vi "think.vi"(0 "X":i8, 1 "Y":i8, 2 "Sensor Array":i8[][](array[numeric]), 3 "Sense Heading":i8, 4 "E":i8) -> (5 "V Heading":i8)   [LabVIEW 2012]
doc: "Chooses a direction of travel based on the direction to the highest-valued block in the world at a given moment. These values are assigned based on known food locations, potential food locations, and proximity to the current robot location."
panel:
  out "Tan":dbl
  out "Expected Value":dbl[][](array[numeric])
  out "Robot Memory":i8[][](array[numeric])
  # "World Key\n-1 = not visited\n0 = no food\n[1...] = food"
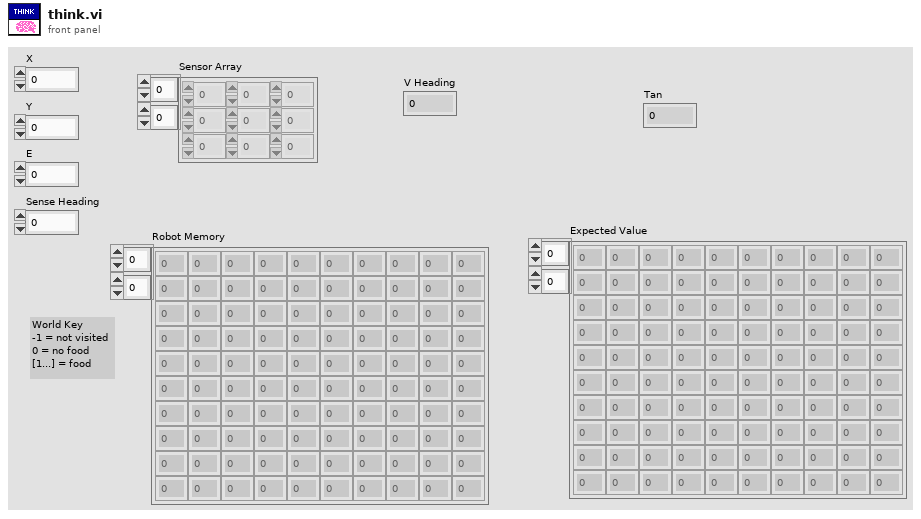
[diagram p1: front panel]
types:
  T1 = cluster{"[0]":i32, "[1]":i32, "[2]":i32, "[3]":i32, "[4]":i32, "[5]":i32, "[6]":i32, "[7]":i32, "[8]":i32}
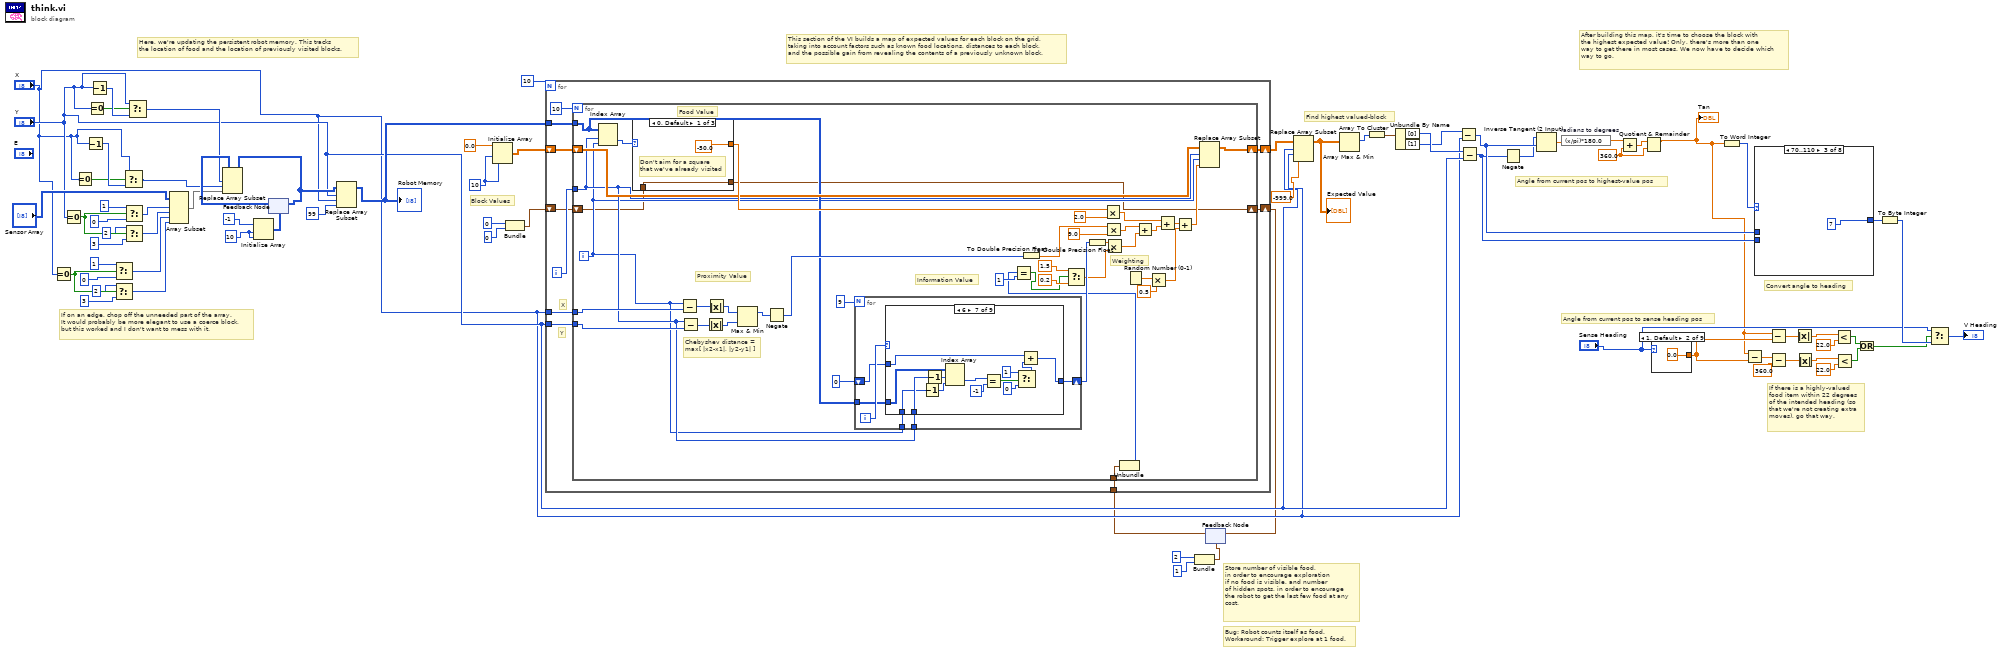
[diagram p0: block diagram]
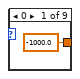
[diagram p2: hidden frame]
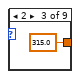
[diagram p3: hidden frame]
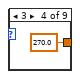
[diagram p4: hidden frame]
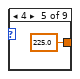
[diagram p5: hidden frame]
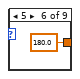
[diagram p6: hidden frame]
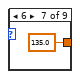
[diagram p7: hidden frame]
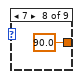
[diagram p8: hidden frame]
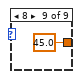
[diagram p9: hidden frame]
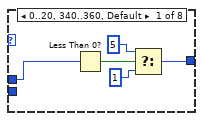
[diagram p10: hidden frame]
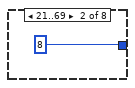
[diagram p11: hidden frame]
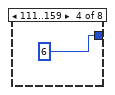
[diagram p12: hidden frame]
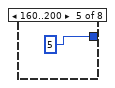
[diagram p13: hidden frame]
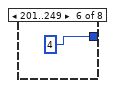
[diagram p14: hidden frame]
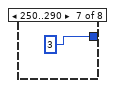
[diagram p15: hidden frame]
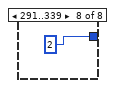
[diagram p16: hidden frame]
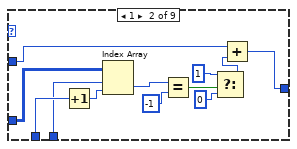
[diagram p18: hidden frame]
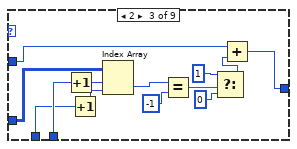
[diagram p19: hidden frame]
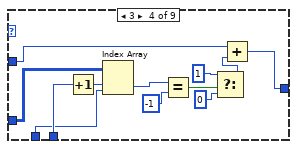
[diagram p20: hidden frame]
diagram:
  w31 = 360.0
  w44 = 10
  w74 = 10
  # "If there is a highly-valued\nfood item within 22 degrees\nof the intended heading (so\nthat we're not creating extra\nmoves), go that way."
  # "Angle from current pos to sense heading pos"
  # "Angle from current pos to highest-value pos"
  # "Convert angle to heading"
  # "Bug: Robot counts itself as food.\nWorkaround: Trigger explore at 1 food."
  # "Store number of visible food,\nin order to encourage exploration\nif no food is visible, and number\nof hidden spots, in order to encourage\nthe robot to get the last few food at any\ncost."
  # "Find highest valued-block"
  # "Here, we're updating the persistent robot memory. This tracks\nthe location of food and the location of previously visited blocks."
  # "After building this map, it's time to choose the block with\nthe highest expected value! Only, there's more than one\nway to get there in most cases. We now have to decide which\nway to go."
  # "This section of the VI builds a map of expected values for each block on the grid, \ntaking into account factors such as known food locations, distances to each block,\nand the possible gain from revealing the contents of a previously unknown block."
  # "Block Values"
  # "If on an edge, chop off the unneeded part of the array.\nIt would probably be more elegant to use a coerce block,\nbut this worked and I don't want to mess with it."
  n1 = Equal To 0?(x="X") -> (x = 0?=w69:bool)
  n2 = Equal To 0?(x="Y") -> (x = 0?=w62:bool)
  n3 = Equal To 0?(x="X") -> (x = 0?=w52:bool)
  n4 = Decrement(x="X") -> (x-1=w53:i8)
  n5 = Equal To 0?(x="Y") -> (x = 0?=w51:bool)
  n6 = Decrement(x="Y") -> (x-1=w55:i8)
  n7 = Select(t=1, s=w69, f=0) -> (s? t:f=w68:i32)
  n8 = Select(t=2, s=w69, f=3) -> (s? t:f=w67:i32)
  n9 = Select(t="X", s=w52, f=w53) -> (s? t:f=w50:i8)
  n10 = Select(t=1, s=w62, f=0) -> (s? t:f=w57:i32)
  n11 = Select(t=2, s=w62, f=3) -> (s? t:f=w56:i32)
  n12 = Select(t="Y", s=w51, f=w55) -> (s? t:f=w54:i8)
  n13 = Array Subset(array="Sensor Array", index (row)=w57, length (row)=w56, index (col)=w68, length (col)=w67) -> (w71:i8[][])
  n14 = Initialize Array(i8 -1, w74, w74) -> (w73:i8[][])
  n15 = feedback #1(w73) -> (w72:i8[][])
  n16 = Replace Array Subset(array=w72, new element=w71, index (row)=w54, index (col)=w50) -> (w49:i8[][])
  n17 = feedback-in #1(w49) -> ()
  n18 = Replace Array Subset(array=w49, new element=i8 99, index (row)="Y", index (col)="X") -> (w47:i8[][])
  "Robot Memory" <- w47
  n19 = Initialize Array(0.0, w44, w44) -> (w46:dbl[][])
  n20 = Bundle(0, 0) -> (w17:cluster{i32, i32})  [unwired: 1 in]
  n21 = Bundle(2, 1) -> (w21:cluster{i32, i32})  [unwired: 1 in]
  n22 = feedback #2(w21) -> (w24:cluster{i32, i32})
  n23 = for {
    N: 10 -> [_]
    tunnel: w47 -> [w85]
    shift-right: [w83] -> w38
    shift-left: w46 -> [w84]
    tunnel: "Y" -> [w80]
    tunnel: "X" -> [w79]
    shift-right: [w77] -> w23
    shift-left: w17 -> [w78]
    tunnel: w24 -> [w76]
    i -> [w81]
    # "Y"
    # "X"
    n24 = for {
      N: 10 -> [_]
      tunnel: w85 -> [w109]
      shift-right: [w121] -> w83
      shift-left: w84 -> [w119]
      tunnel: w81 -> [w102]
      tunnel: w80 -> [w107]
      tunnel: w79 -> [w108]
      shift-right: [w99] -> w77
      shift-left: w78 -> [w100]
      tunnel: w76 -> [w87]
      i -> [w101]
      # "Chebyshev distance =\nmax[ |x2-x1|, |y2-y1| ]"
      # "Information Value"
      # "Weighting"
      # "Proximity Value"
      # "Food Value"
      n25 = Index Array(array=w109, index (row)=w102, index (col)=w101) -> (element=w125:i8)
      n26 = case shown="0, Default" w125 {
        selector: w125 -> [_ w240 _]
        tunnel: [-50.0 w241 0.5] -> w122
        tunnel: w100 -> [w233 w238 w245]
        tunnel: [w233 w239 w246] -> w99
        frame 0, Default {
          # "Don't aim for a square\nthat we've already visited"
        }
        frame 1.. {
          n27 = Unbundle(w238) -> (w236:i32, w235:i32)
          n28 = Increment(x=w236) -> (x+1=w237:i32)
          n29 = To Double Precision Float(number=w240) -> (double precision float=w241:dbl)
          n30 = Bundle(w237, w235) -> (w239:cluster{i32, i32})  [unwired: 1 in]
        }
        frame -1 {
          n31 = Unbundle(w245) -> (w242:i32, w243:i32)
          n32 = Increment(x=w243) -> (x+1=w244:i32)
          n33 = Bundle(w242, w244) -> (w246:cluster{i32, i32})  [unwired: 1 in]
        }
      }
      n34 = Subtract(x=w101, y=w108) -> (x-y=w118:i32)
      n35 = Subtract(x=w102, y=w107) -> (x-y=w117:i32)
      n36 = Absolute Value(x=w117) -> (abs(x)=w116:i32)
      n37 = Absolute Value(x=w118) -> (abs(x)=w115:i32)
      n38 = Max & Min(x=w115, y=w116) -> (max(x,y)=w114:i32)  [unwired: 1 out]
      n39 = Negate(x=w114) -> (-x=w112:i32)
      n40 = for {
        N: 9 -> [_]
        shift-right: [w129] -> w103
        shift-left: 0 -> [w130]
        tunnel: w109 -> [w128]
        tunnel: w101 -> [w127]
        tunnel: w102 -> [w126]
        i -> [w131]
        n41 = case shown="6" w131 {
          tunnel: w130 -> [w132 w142 w155 w167 w180 w192 w205 w217 w230]
          tunnel: [w132 w141 w154 w166 w179 w191 w204 w216 w229] -> w129
          tunnel: w128 -> [_ w144 w157 w169 w182 w194 w207 w219 w232]
          tunnel: w127 -> [_ w134 w145 w158 w172 w184 w197 w208 w221]
          tunnel: w126 -> [_ w133 w146 w160 w170 w183 w198 w209 w223]
          frame 0, Default {
          }
          frame 1 {
            n42 = Increment(x=w134) -> (x+1=w135:i32)
            n43 = Index Array(array=w144, index (row)=w133, index (col)=w135) -> (element=w137:i8)
            n44 = Equal?(x=w137, y=i8 -1) -> (x = y?=w138:bool)
            n45 = Select(t=1, s=w138, f=0) -> (s? t:f=w143:i32)
            n46 = Add(x=w142, y=w143) -> (x+y=w141:i32)
          }
          frame 2 {
            n47 = Increment(x=w146) -> (x+1=w147:i32)
            n48 = Increment(x=w145) -> (x+1=w148:i32)
            n49 = Index Array(array=w157, index (row)=w147, index (col)=w148) -> (element=w150:i8)
            n50 = Equal?(x=w150, y=i8 -1) -> (x = y?=w151:bool)
            n51 = Select(t=1, s=w151, f=0) -> (s? t:f=w156:i32)
            n52 = Add(x=w155, y=w156) -> (x+y=w154:i32)
          }
          frame 3 {
            n53 = Increment(x=w160) -> (x+1=w159:i32)
            n54 = Index Array(array=w169, index (row)=w159, index (col)=w158) -> (element=w162:i8)
            n55 = Equal?(x=w162, y=i8 -1) -> (x = y?=w163:bool)
            n56 = Select(t=1, s=w163, f=0) -> (s? t:f=w168:i32)
            n57 = Add(x=w167, y=w168) -> (x+y=w166:i32)
          }
          frame 4 {
            n58 = Increment(x=w170) -> (x+1=w171:i32)
            n59 = Decrement(x=w172) -> (x-1=w173:i32)
            n60 = Index Array(array=w182, index (row)=w171, index (col)=w173) -> (element=w175:i8)
            n61 = Equal?(x=w175, y=i8 -1) -> (x = y?=w176:bool)
            n62 = Select(t=1, s=w176, f=0) -> (s? t:f=w181:i32)
            n63 = Add(x=w180, y=w181) -> (x+y=w179:i32)
          }
          frame 5 {
            n64 = Decrement(x=w184) -> (x-1=w185:i32)
            n65 = Index Array(array=w194, index (row)=w183, index (col)=w185) -> (element=w187:i8)
            n66 = Equal?(x=w187, y=i8 -1) -> (x = y?=w188:bool)
            n67 = Select(t=1, s=w188, f=0) -> (s? t:f=w193:i32)
            n68 = Add(x=w192, y=w193) -> (x+y=w191:i32)
          }
          frame 6 {
            n69 = Decrement(x=w197) -> (x-1=w195:i32)
            n70 = Decrement(x=w198) -> (x-1=w196:i32)
            n71 = Index Array(array=w207, index (row)=w196, index (col)=w195) -> (element=w200:i8)
            n72 = Equal?(x=w200, y=i8 -1) -> (x = y?=w201:bool)
            n73 = Select(t=1, s=w201, f=0) -> (s? t:f=w206:i32)
            n74 = Add(x=w205, y=w206) -> (x+y=w204:i32)
          }
          frame 7 {
            n75 = Decrement(x=w209) -> (x-1=w210:i32)
            n76 = Index Array(array=w219, index (row)=w210, index (col)=w208) -> (element=w212:i8)
            n77 = Equal?(x=w212, y=i8 -1) -> (x = y?=w213:bool)
            n78 = Select(t=1, s=w213, f=0) -> (s? t:f=w218:i32)
            n79 = Add(x=w217, y=w218) -> (x+y=w216:i32)
          }
          frame 8 {
            n80 = Increment(x=w221) -> (x+1=w222:i32)
            n81 = Decrement(x=w223) -> (x-1=w220:i32)
            n82 = Index Array(array=w232, index (row)=w220, index (col)=w222) -> (element=w225:i8)
            n83 = Equal?(x=w225, y=i8 -1) -> (x = y?=w226:bool)
            n84 = Select(t=1, s=w226, f=0) -> (s? t:f=w231:i32)
            n85 = Add(x=w230, y=w231) -> (x+y=w229:i32)
          }
        }
      }
      n86 = To Double Precision Float(number=w112) -> (double precision float=w113:dbl)
      n87 = To Double Precision Float(number=w103) -> (double precision float=w104:dbl)
      n88 = Multiply(x=w122, y=2.0) -> (x*y=w93:dbl)
      n89 = Multiply(x=w113, y=9.0) -> (x*y=w124:dbl)
      n90 = Unbundle(w87) -> (w86:i32)  [unwired: 1 out]
      n91 = Equal?(x=w86, y=1) -> (x = y?=w95:bool)
      n92 = Select(t=1.5, s=w95, f=0.2) -> (s? t:f=w96:dbl)
      n93 = Multiply(x=w104, y=w96) -> (x*y=w123:dbl)
      n94 = Random Number (0-1)() -> (number: 0 to 1=w90:dbl)
      n95 = Add(x=w124, y=w123) -> (x+y=w92:dbl)
      n96 = Multiply(x=w90, y=0.5) -> (x*y=w89:dbl)
      n97 = Add(x=w93, y=w92) -> (x+y=w91:dbl)
      n98 = Add(x=w91, y=w89) -> (x+y=w120:dbl)
      n99 = Replace Array Subset(array=w119, new element=w120, index (row)=w102, index (col)=w101) -> (w121:dbl[][])
    }
  }
  n100 = feedback-in #2(w23) -> ()
  n101 = Replace Array Subset(array=w38, new element=-999.0, index (row)="Y", index (col)="X") -> (w34:dbl[][])
  "Expected Value" <- w34
  n102 = Array Max & Min(array=w34) -> (max index (indices)=w42:i32[])  [unwired: 3 out]
  n103 = Array To Cluster(array=w42) -> (cluster=w41:T1)
  n104 = Unbundle By Name(w41) -> ("[0]"=w40:i32, "[1]"=w39:i32)
  n105 = Subtract(x=w39, y="X") -> (x-y=w28:i32)
  n106 = Subtract(x=w40, y="Y") -> (x-y=w26:i32)
  n107 = Negate(x=w26) -> (-x=w27:i32)
  n108 = Inverse Tangent (2 Input)(1:w28, 2:w27) -> (0:w29:dbl)
  n109 = expression code="(x/pi)*180.0" "radians to degrees"(w29) -> (w33:dbl)
  n110 = Add(x=w33, y=w31) -> (x+y=w32:dbl)
  n111 = Quotient & Remainder(x=w32, y=w31) -> (x-y*floor(x/y)=w2:dbl)  [unwired: 1 out]
  "Tan" <- w2
  n112 = case shown="1, Default" "Sense Heading" {
    tunnel: [-1000.0 0.0 315.0 270.0 225.0 180.0 135.0 90.0 45.0] -> w3
    frame 0 {
    }
    frame 1, Default {
    }
    frame 2 {
    }
    frame 3 {
    }
    frame 4 {
    }
    frame 5 {
    }
    frame 6 {
    }
    frame 7 {
    }
    frame 8 {
    }
  }
  n113 = To Word Integer(number=w2) -> (16bit integer=w30:i16)
  n114 = Subtract(x=w2, y=w3) -> (x-y=w5:dbl)
  n115 = case shown="70..110" w30 {
    tunnel: w28 -> [w258 _ _ _ _ _ _ _]
    tunnel: w26 -> [_ _ _ _ _ _ _ _]
    tunnel: [w257 8 7 6 5 4 3 2] -> w25
    frame 0..20, 340..360, Default {
      n116 = Less Than 0?(x=w258) -> (x < 0?=w259:bool)
      n117 = Select(t=5, s=w259, f=1) -> (s? t:f=w257:i32)
    }
    frame 21..69 {
    }
    frame 70..110 {
    }
    frame 111..159 {
    }
    frame 160..200 {
    }
    frame 201..249 {
    }
    frame 250..290 {
    }
    frame 291..339 {
    }
  }
  n118 = Subtract(x=w2, y=w3) -> (x-y=w7:dbl)
  n119 = Subtract(x=w5, y=360.0) -> (x-y=w6:dbl)
  n120 = Absolute Value(x=w7) -> (abs(x)=w15:dbl)
  n121 = Absolute Value(x=w6) -> (abs(x)=w1:dbl)
  n122 = Less?(x=w15, y=22.0) -> (x < y?=w11:bool)
  n123 = Less?(x=w1, y=22.0) -> (x < y?=w8:bool)
  n124 = Or(x=w11, y=w8) -> (x .or. y?=w10:bool)
  n125 = To Byte Integer(number=w25) -> (8bit integer=w13:i8)
  n126 = Select(t="Sense Heading", s=w10, f=w13) -> (s? t:f=→"V Heading":i8)
